vi "Trigger IMAQ.vi"() -> ()   [LabVIEW 2012]
panel:
  in  "ICImagingControl":refnum<k7>(container)
  in  "Open Device Configuration (Monochrome  Images)":bool
  in  "Open Device Configuration (Color Images)":bool
  out "ReferenceTimeStart":dbl
  out "Image Age":dbl
  out "ReferenceTimeCurrent":dbl
  out "SampleStartTime":dbl
  in  "External Trigger":bool
  in  "Grab":bool
  in  "End Program":bool
  # "Open Device Configuration"
  # "Off"
  # "On"
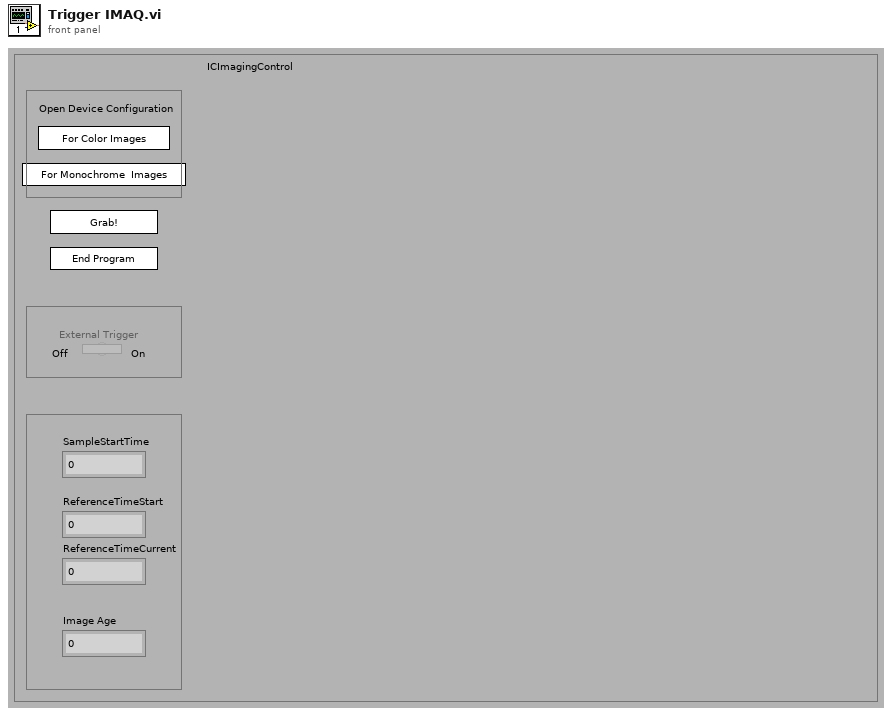
[diagram p1: front panel]
types:
  T1 = typedef "IMAQ Image.ctl" = refnum<image>
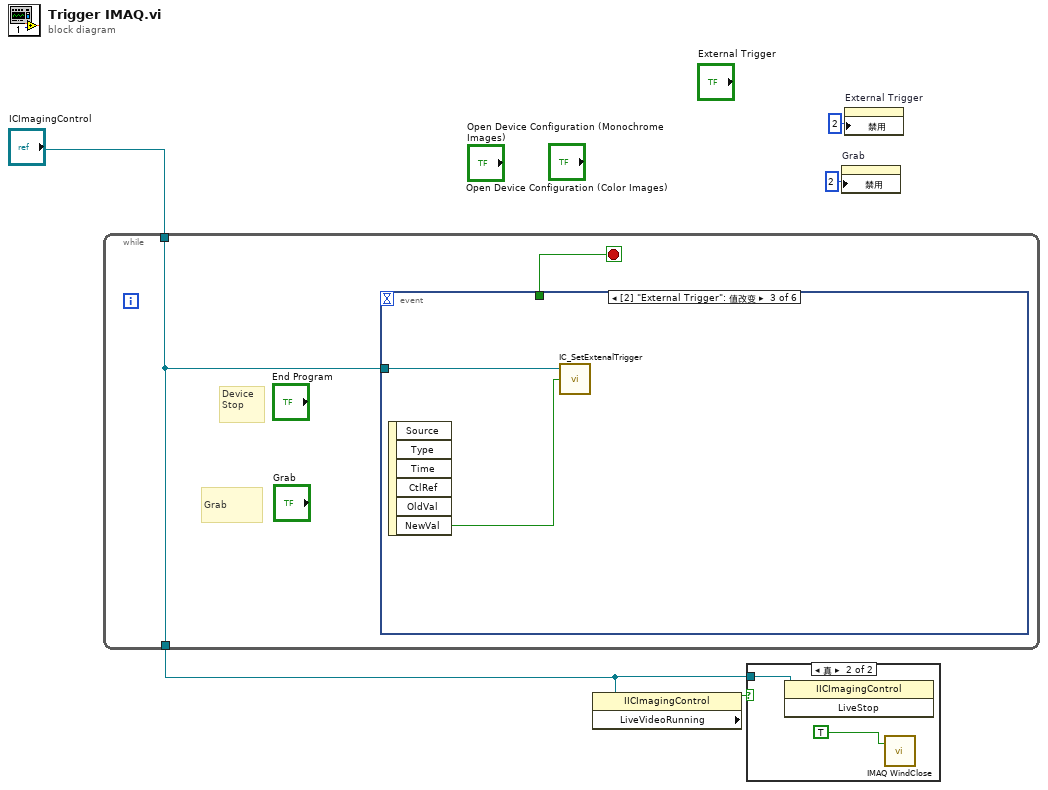
[diagram p0: block diagram]
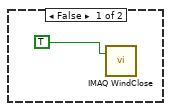
[diagram p2: hidden frame]
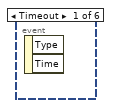
[diagram p3: hidden frame]
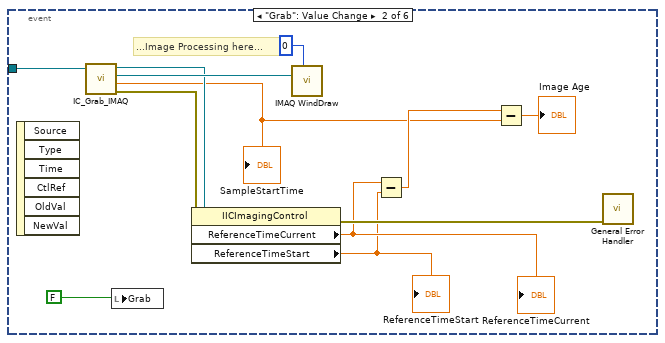
[diagram p4: hidden frame]
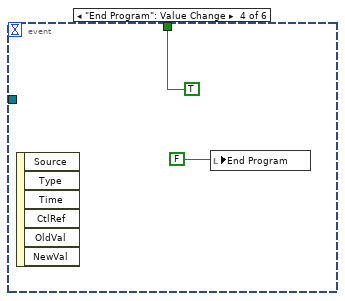
[diagram p5: hidden frame]
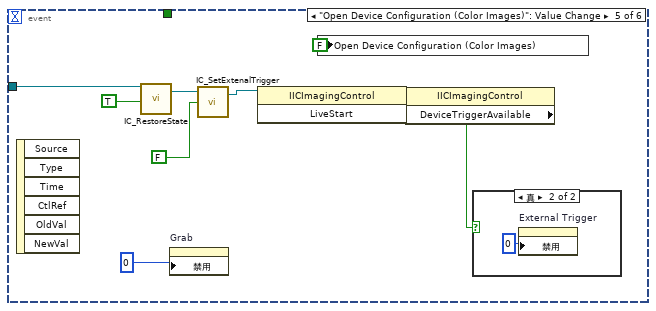
[diagram p6: hidden frame]
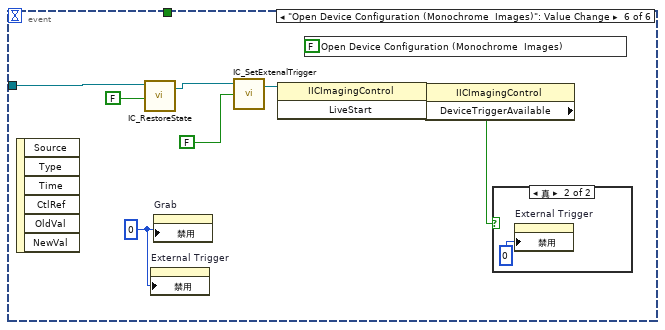
[diagram p8: hidden frame]
diagram:
  n1 = while {
    tunnel: "ICImagingControl" -> [w6]
    tunnel: [w6] -> w4
    stop <- w7 stop-if-true
    # "Device\nStop"
    # "Grab"
    n2 = event shown="[2] \"External Trigger\": 值改变" {
      selector: _ -> [_ _ _ _ _ _]
      dyn-events: _ -> [_ _ _ _ _ _]
      timeout: _ -> [_ _ _ _ _ _]
      tunnel: w6 -> [_ w17 w21 _ w32 w41]
      tunnel: [_ _ _ TRUE _ _] -> w7
      event Timeout {
        n3 = event-data() -> ()  [unwired: 1 in, 2 out]
      }
      event "Grab": Value Change {
        # "...Image Processing here..."
        n4 = event-data() -> ()  [unwired: 1 in, 6 out]
        n5 = call "IC_Grab_IMAQ.vi"("ICImagingControl In"=w17) -> ("ICImagingControl Out"=w15:refnum<k7>, "Image Out"=w16:T1, "SampleStartTime"=w10:dbl, "Error Out"=w12:errorcluster)  [unwired: 2 in]
        "SampleStartTime" <- w10
        n6 = local write "Grab"(FALSE) -> ()
        n7 = property class="IICImagingControl"(reference=w15, error in=w12) -> (error out=w13:errorcluster, "ReferenceTimeCurrent"=w9:dbl, "ReferenceTimeStart"=w8:dbl)  [unwired: 1 out]
        "ReferenceTimeCurrent" <- w9
        "ReferenceTimeStart" <- w8
        n8 = call "IMAQ WindDraw"("Window Number (0...15)"=0, "Image"=w16) -> ()  [unwired: 8 in, 2 out]
        n9 = Subtract(x=w9, y=w8) -> (x-y=w11:dbl)
        n10 = Subtract(x=w11, y=w10) -> (x-y=→"Image Age":dbl)
        n11 = call <vilib>:"General Error Handler.vi"("error in (no error)"=w13) -> ()  [unwired: 10 in, 5 out]
      }
      event "External Trigger": Value Change {
        n12 = event-data() -> ("NewVal"=w20:bool)  [unwired: 1 in, 5 out]
        n13 = call <userlib>:"IC_SetExtenalTrigger.vi"("Trigger"=w20, "ICImagingControl In"=w21) -> ()  [unwired: 1 in, 2 out]
      }
      event "End Program": Value Change {
        n14 = event-data() -> ()  [unwired: 1 in, 6 out]
        n15 = local write "End Program"(FALSE) -> ()
      }
      event "Open Device Configuration (Color Images)": Value Change {
        n16 = event-data() -> ()  [unwired: 1 in, 6 out]
        n17 = call "IC_RestoreState.vi"("Color"=TRUE, "ICImagingControl"=w32) -> ("ICImagingControl Out"=w24:refnum<k7>)  [unwired: 2 in, 1 out]
        n18 = property on="Grab" class="Bool (严格)"("禁用"=0) -> ()  [unwired: 2 in, 2 out]
        n19 = call <userlib>:"IC_SetExtenalTrigger.vi"("Trigger"=FALSE, "ICImagingControl In"=w24) -> ("ICImagingControl Out"=w25:refnum<k7>)  [unwired: 1 in, 1 out]
        n20 = invoke class="IICImagingControl" method="LiveStart"(reference=w25) -> (reference out=w27:refnum<k7>)  [unwired: 2 in, 2 out]
        n21 = local write "Open Device Configuration (Color Images)"(FALSE ("Open Device Configuration (Color Images)")) -> ()
        n22 = property class="IICImagingControl"(reference=w27) -> ("DeviceTriggerAvailable"=w26:bool)  [unwired: 1 in, 2 out]
        n23 = case shown="真" w26 {
          frame False {
          }
          frame True {
            n24 = property on="External Trigger" class="Bool (严格)"("禁用"=u8 0 ("Disabled")) -> ()  [unwired: 2 in, 2 out]
          }
        }
      }
      event "Open Device Configuration (Monochrome  Images)": Value Change {
        w39 = 0
        n25 = event-data() -> ()  [unwired: 1 in, 6 out]
        n26 = call "IC_RestoreState.vi"("Color"=FALSE, "ICImagingControl"=w41) -> ("ICImagingControl Out"=w34:refnum<k7>)  [unwired: 2 in, 1 out]
        n27 = property on="External Trigger" class="Bool (严格)"("禁用"=w39) -> ()  [unwired: 2 in, 2 out]
        n28 = property on="Grab" class="Bool (严格)"("禁用"=w39) -> ()  [unwired: 2 in, 2 out]
        n29 = call <userlib>:"IC_SetExtenalTrigger.vi"("Trigger"=FALSE, "ICImagingControl In"=w34) -> ("ICImagingControl Out"=w37:refnum<k7>)  [unwired: 1 in, 1 out]
        n30 = invoke class="IICImagingControl" method="LiveStart"(reference=w37) -> (reference out=w36:refnum<k7>)  [unwired: 2 in, 2 out]
        n31 = local write "Open Device Configuration (Monochrome  Images)"(FALSE ("Open Device Configuration (Monochrome  Images)")) -> ()
        n32 = property class="IICImagingControl"(reference=w36) -> ("DeviceTriggerAvailable"=w35:bool)  [unwired: 1 in, 2 out]
        n33 = case shown="真" w35 {
          frame False {
          }
          frame True {
            n34 = property on="External Trigger" class="Bool (严格)"("禁用"=u8 0 ("Disabled")) -> ()  [unwired: 2 in, 2 out]
          }
        }
      }
    }
  }
  n35 = property class="IICImagingControl"(reference=w4) -> ("LiveVideoRunning"=w5:bool)  [unwired: 1 in, 2 out]
  n36 = case shown="真" w5 {
    tunnel: w4 -> [_ w46]
    frame False {
      n37 = call "IMAQ WindClose"("Close All Windows (False)"=TRUE) -> ()  [unwired: 5 in, 1 out]
    }
    frame True {
      n38 = invoke class="IICImagingControl" method="LiveStop"(reference=w46) -> ()  [unwired: 2 in, 3 out]
      n39 = call "IMAQ WindClose"("Close All Windows (False)"=TRUE) -> ()  [unwired: 5 in, 1 out]
    }
  }
  n40 = property on="Grab" class="Bool (严格)"("禁用"=u8 2 ("Disabled")) -> ()  [unwired: 2 in, 2 out]
  n41 = property on="External Trigger" class="Bool (严格)"("禁用"=u8 2 ("Disabled")) -> ()  [unwired: 2 in, 2 out]
